vi "Get Output Pct.vi"(8 "error in (no error)":errorcluster, 11 "Pump in":refnum<class "Pump.lvclass">) -> (0 "error out":errorcluster, 2 "Output %":dbl, 3 "Pump out":refnum<class "Pump.lvclass">)   [LabVIEW 2014, in "Pump.lvclass"]
uses:
  Pump.lvclass
  Pump.lvclass/Pump.ctl
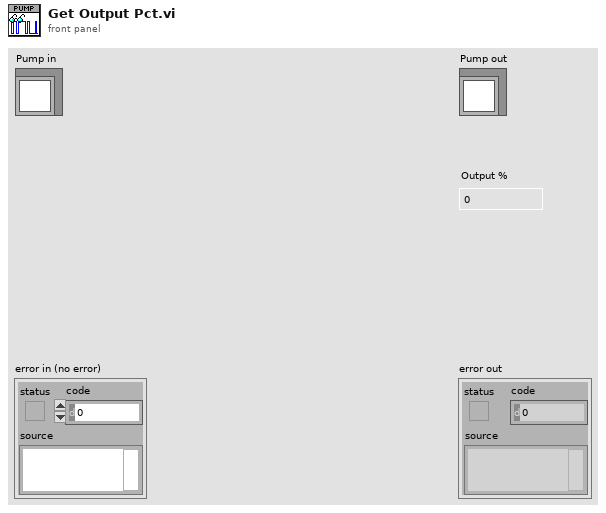
[diagram p1: front panel]
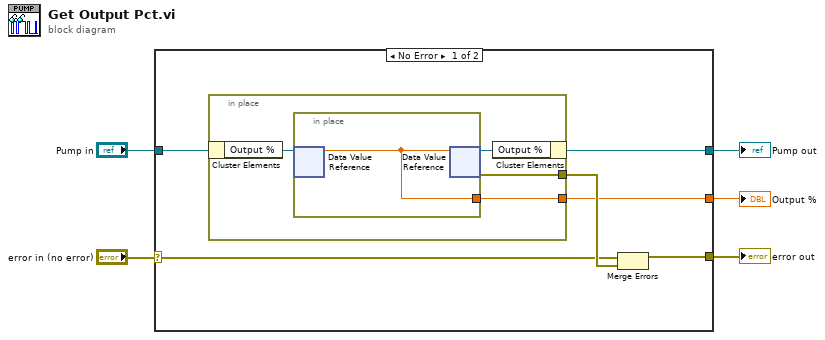
[diagram p0: block diagram]
diagram:
  n1 = case shown="No Error" "error in (no error)" {
    selector: "error in (no error)" -> [w8 w18]
    tunnel: [w7 w18] -> w4
    tunnel: [w10 w17] -> w2
    tunnel: "Pump in" -> [w11 w17]
    tunnel: [w6 _] -> w1
    frame No Error {
      n2 = in-place {
        in-place-border: [w13] -> w9
        in-place-border: [w12] -> w6
        n3 = in-place-cluster #1(w11) -> ("Output %"=w15:refnum<data-value>)
        n4 = in-place {
          in-place-border: [w16] -> w12
          n5 = in-place-dvr #2(w15) -> (w16:dbl)  [unwired: 1 out]
          n6 = in-place-dvr #2(w16) -> (w14:refnum<data-value>, w13:errorcluster)
        }
        n7 = in-place-cluster #1("Output %"=w14) -> (w10:refnum<class "Pump.lvclass">)
      }
      n8 = Merge Errors(w8, w9) -> (w7:errorcluster)
    }
    frame Error {
    }
  }
  "error out" <- w4
  "Pump out" <- w2
  "Output %" <- w1
